vi "Write Parent Chromosomes.vi"(8 "error in (no error)":errorcluster, 10 "Chromosomes":refnum<data-value>, 11 "IPopulation in":refnum<class "IPopulation.lvclass">) -> (0 "error out":errorcluster, 3 "IPopulation out":refnum<class "IPopulation.lvclass">)   [LabVIEW 2016, in "IPopulation.lvclass"]
uses:
  IPopulation.lvclass
  IChromosome/IChromosome.lvclass
  IPopulation.lvclass/IPopulation.ctl
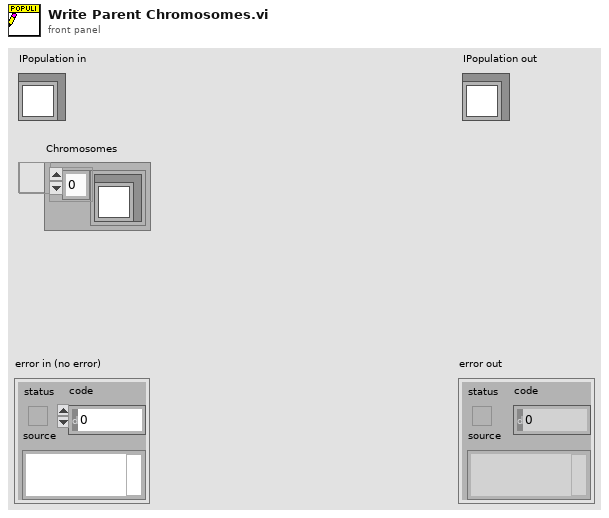
[diagram p1: front panel]
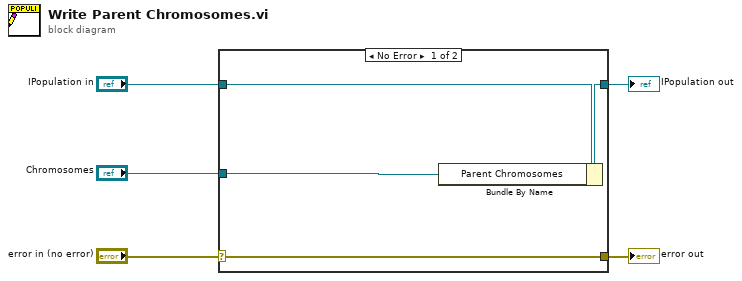
[diagram p0: block diagram]
diagram:
  n1 = case shown="No Error" "error in (no error)" {
    selector: "error in (no error)" -> [w9 w10]
    tunnel: [w9 w10] -> w4
    tunnel: [w7 w11] -> w2
    tunnel: "IPopulation in" -> [w8 w11]
    tunnel: "Chromosomes" -> [w6 _]
    frame No Error {
      n2 = Bundle By Name(cluster=w8, "Parent Chromosomes"=w6) -> (w7:refnum<class "IPopulation.lvclass">)
    }
    frame Error {
    }
  }
  "error out" <- w4
  "IPopulation out" <- w2
